vi "Write 7z.bat.vi"(8 "error in (no error)":errorcluster, 11 "PostBuildSupport in":refnum<class "PostBuildSupport.lvclass">) -> (0 "error out":errorcluster, 3 "PostBuildSupport out":refnum<class "PostBuildSupport.lvclass">)   [LabVIEW 2019, in "PostBuildSupport.lvclass"]
uses:
  PostBuildSupport.lvclass
  PostBuildSupport.lvclass/PostBuildSupport.ctl
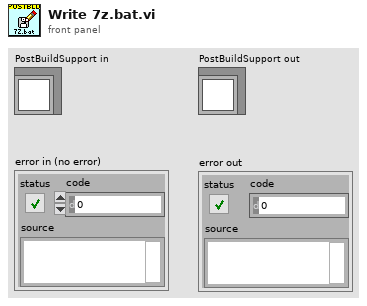
[diagram p1: front panel]
types:
  T1 = enum16{"open", "replace", "create", "open or create", "replace or create", "replace or create with confirmation"}
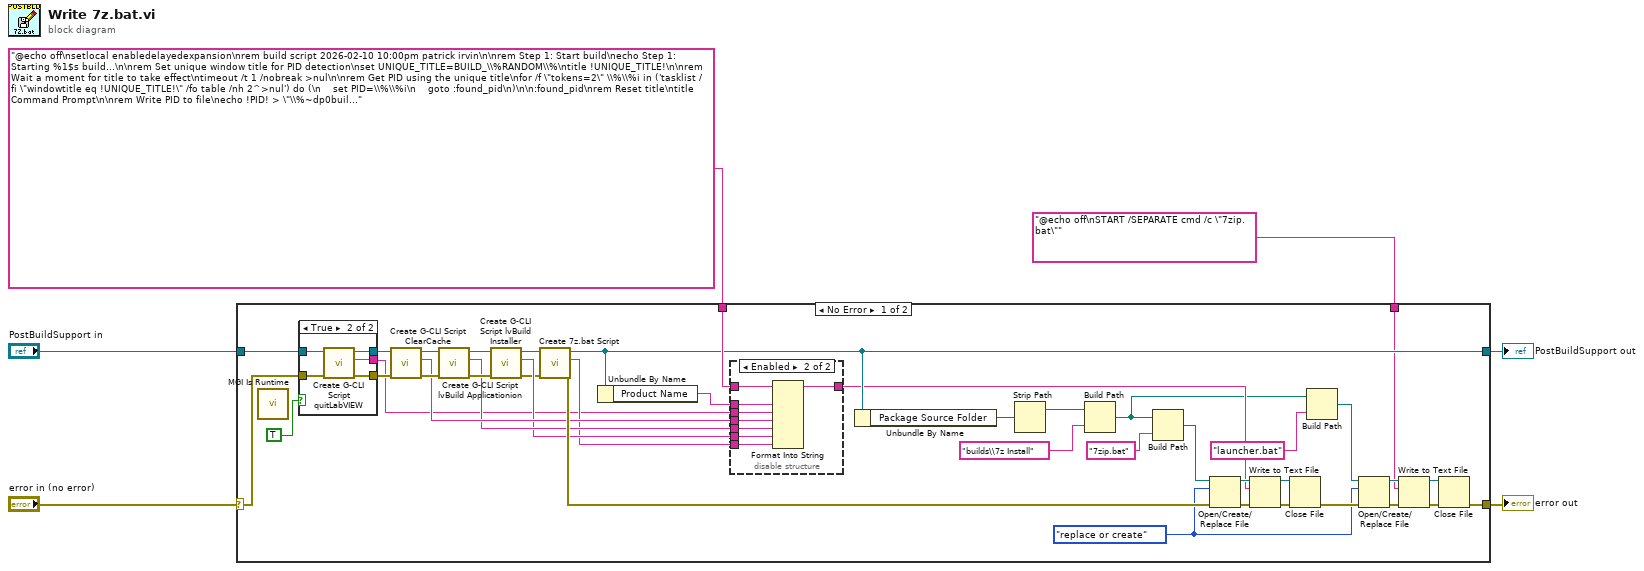
[diagram p0: block diagram]
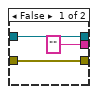
[diagram p2: hidden frame]
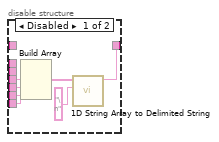
[diagram p3: hidden frame]
diagram:
  n1 = case shown="No Error" "error in (no error)" {
    selector: "error in (no error)" -> [w28 w72]
    tunnel: [w14 w72] -> w6
    tunnel: "PostBuildSupport in" -> [w30 w71]
    tunnel: [w23 w71] -> w3
    tunnel: "@echo off\nsetlocal enabledelayedexpansion\nrem build script 2026-02-10 10:00pm patrick irvin\n\nrem Step 1: Start build\necho Step 1: Starting %1$s build...\n\nrem Set unique window title for PID detection\nset UNIQUE_TITLE=BUILD_\\%RANDOM\\%\ntitle !UNIQUE_TITLE!\n\nrem Wait a moment for title to take effect\ntimeout /t 1 /nobreak >nul\n\nrem Get PID using the unique title\nfor /f \"tokens=2\" \\%\\%i in ('tasklist /fi \"windowtitle eq !UNIQUE_TITLE!\" /fo table /nh 2^>nul') do (\n    set PID=\\%\\%i\n    goto :found_pid\n)\n\n:found_pid\nrem Reset title\ntitle Command Prompt\n\nrem Write PID to file\necho !PID! > \"\\%~dp0build_pid.txt\"\necho Found PID: !PID!\n\nrem Test PID detection (only if PID is not empty)\nif not \"!PID!\"==\"\" (\n    echo Testing PID !PID!:\n    tasklist /fi \"PID eq !PID!\" /nh\n) else (\n    echo Warning: Could not determine PID\n)\n\nrem Initialize status\necho RUNNING,\\%TIME\\%,Getting PID... > \"\\%~dp0build_status.txt\"\ntimeout /t 1 /nobreak >nul\n\necho RUNNING,\\%TIME\\%,PID=!PID! detected > \"\\%~dp0build_status.txt\"\ntimeout /t 1 /nobreak >nul\n\nrem Step 2: Quit LabVIEW\necho Step 2: Quitting LabVIEW...\necho RUNNING,\\%TIME\\%,Step 2 - Quitting LabVIEW > \"\\%~dp0build_status.txt\"\n%2$s\nif !errorlevel! neq 0 (\n    echo ERROR,\\%TIME\\%,Step 2 failed - Quitting LabVIEW failed > \"\\%~dp0build_status.txt\"\n    goto :error_exit\n)\n\nrem Step 3: Clear Cache\necho Step 3: Clearing cache...\necho RUNNING,\\%TIME\\%,Step 3 - Clearing cache > \"\\%~dp0build_status.txt\"\n%3$s\nif !errorlevel! neq 0 (\n    echo ERROR,\\%TIME\\%,Step 3 failed - Cache clearing failed > \"\\%~dp0build_status.txt\"\n    goto :error_exit\n)\n\nrem Step 4: Build Application\necho Step 4: Building application...\necho RUNNING,\\%TIME\\%,Step 4 - Building application > \"\\%~dp0build_status.txt\"\n%4$s\nif !errorlevel! neq 0 (\n    echo ERROR,\\%TIME\\%,Step 4 failed - Application build failed > \\%%~dp0build_status.txt\"\n    goto :error_exit\n)\n\nrem Step 5: Build Installer\necho Step 5: Building installer...\necho RUNNING,\\%TIME\\%,Step 5 - Building installer > \"\\%~dp0build_status.txt\"\n%5$s\nif !errorlevel! neq 0 (\n    echo ERROR,\\%TIME\\%,Step 5 failed - Installer build failed > \"\\%~dp0build_status.txt\"\n    goto :error_exit\n)\n\nrem Step 6: Creating 7z archive and self-extracting installer\necho Step 6: Creating 7z archive and self-extracting installer...\necho RUNNING,\\%TIME\\%,Step 6 - Creating 7z archive and self-extracting installer > \"\\%~dp0build_status.txt\"\n%6$s\nif !errorlevel! neq 0 (\n    echo ERROR,\\%TIME\\%,Step 6 failed - 7z archive creation failed > \"\\%~dp0build_status.txt\"\n    goto :error_exit\n)\n\nrem Success - Update final status\necho SUCCESS,\\%TIME\\%,Build completed successfully! > \"\\%~dp0build_status.txt\"\necho Build process finished successfully. (PID=!PID!)\ngoto :end\n\n:error_exit\necho Build process failed. Check \"\\%~dp0build_status.txt\" for details. (PID=!PID!)\nexit /b 1\n\n:end" ("name or relative path") -> [w25 _]
    tunnel: "@echo off\nSTART /SEPARATE cmd /c \"7zip.bat\"" ("name or relative path") -> [w13 _]
    frame No Error {
      w9 = T1."replace or create" ("operation (0:open)")
      n2 = call <userlib>:"MGI Is Runtime.vi"() -> ()  [unwired: 7 in, 1 out]
      n3 = case shown="True" TRUE {
        tunnel: [w50 w55] -> w32
        tunnel: [w48 w54] -> w31
        tunnel: w28 -> [w48 w53]
        tunnel: w30 -> [w50 w52]
        tunnel: ["" ("command") w51] -> w22
        frame False {
        }
        frame True {
          n4 = call "Create G-CLI Script quitLabVIEW.vi"("error in (no error)"=w53, "PostBuildSupport in"=w52) -> ("error out"=w54:errorcluster, "command"=w51:string, "PostBuildSupport out"=w55:refnum<class "PostBuildSupport.lvclass">)  [unwired: 7 in]
        }
      }
      n5 = call "Create G-CLI Script ClearCache.vi"("error in (no error)"=w31, "PostBuildSupport in"=w32) -> ("error out"=w39:errorcluster, "command"=w35:string, "PostBuildSupport out"=w38:refnum<class "PostBuildSupport.lvclass">)  [unwired: 7 in]
      n6 = call "Create G-CLI Script lvBuild Applicationion.vi"("error in (no error)"=w39, "PostBuildSupport in"=w38) -> ("error out"=w36:errorcluster, "command"=w34:string, "PostBuildSupport out"=w37:refnum<class "PostBuildSupport.lvclass">)  [unwired: 7 in]
      n7 = call "Create G-CLI Script lvBuild Installer.vi"("error in (no error)"=w36, "PostBuildSupport in"=w37) -> ("error out"=w26:errorcluster, "command"=w33:string, "PostBuildSupport out"=w27:refnum<class "PostBuildSupport.lvclass">)  [unwired: 7 in]
      n8 = call "Create 7z.bat Script.vi"("error in (no error)"=w26, "PostBuildSupport in"=w27) -> ("error out"=w44:errorcluster, "resulting string"=w29:string, "PostBuildSupport out"=w23:refnum<class "PostBuildSupport.lvclass">)  [unwired: 7 in]
      n9 = Unbundle By Name(w23) -> ("Product Name"=w24:string)
      n10 = disable-structure shown="Enabled" {
        disable-tunnel: w35 -> [w62 w69]
        disable-tunnel: w34 -> [w61 w68]
        disable-tunnel: w33 -> [w60 w67]
        disable-tunnel: w29 -> [w57 w66]
        disable-tunnel: [w56 w65] -> w20
        disable-tunnel: w25 -> [_ w70]
        disable-tunnel: w24 -> [_ w64]
        disable-tunnel: w22 -> [_ w63]
        frame Disabled {
          n11 = Build Array(w62, w61, w60, w57) -> (w59:string[])  [unwired: 1 in]
          n12 = call <vilib>:"1D String Array to Delimited String.vi"("delimiter"="\n", "string array"=w59) -> ("delimited string"=w56:string)  [unwired: 9 in]
        }
        frame Enabled {
          n13 = Format Into String(format string=w70, w64, w63, w69, w68, w67, w66) -> (resulting string=w65:string)  [unwired: 2 in, 1 out]
        }
      }
      n14 = Unbundle By Name(w23) -> ("Package Source Folder"=w46:path)
      n15 = Strip Path(path=w46) -> (stripped path=w47:path)  [unwired: 1 out]
      n16 = Build Path(base path=w47, name or relative path="builds\\7z Install") -> (appended path=w11:path)
      n17 = Build Path(base path=w11, name or relative path="7zip.bat") -> (appended path=w8:path)
      n18 = Open/Create/Replace File(file path (use dialog)=w8, error in=w44, operation (0:open)=w9) -> (refnum out=w43:refnum<file>, error out=w42:errorcluster)  [unwired: 3 in, 1 out]
      n19 = Write to Text File(file (use dialog)=w43, text=w20, error in=w42) -> (refnum out=w40:refnum<file>, error out=w41:errorcluster)  [unwired: 1 in, 1 out]
      n20 = Close File(refnum=w40, error in=w41) -> (error out=w15:errorcluster)  [unwired: 1 out]
      n21 = Build Path(base path=w11, name or relative path="launcher.bat") -> (appended path=w10:path)
      n22 = Open/Create/Replace File(file path (use dialog)=w10, error in=w15, operation (0:open)=w9) -> (refnum out=w16:refnum<file>, error out=w17:errorcluster)  [unwired: 3 in, 1 out]
      n23 = Write to Text File(file (use dialog)=w16, text=w13, error in=w17) -> (refnum out=w19:refnum<file>, error out=w18:errorcluster)  [unwired: 1 in, 1 out]
      n24 = Close File(refnum=w19, error in=w18) -> (error out=w14:errorcluster)  [unwired: 1 out]
    }
    frame Error {
    }
  }
  "error out" <- w6
  "PostBuildSupport out" <- w3
